vi "CRIO_TCPWriteState.vi"(6 "Curr State":T1, 8 "error in (no error)":errorcluster, 9 "Transition? in":bool, 10 "Connected?":bool, 11 "TCP Network Connection in":refnum<k5>) -> (0 "error out":errorcluster, 3 "TCP Network Connection out":refnum<k5>)   [LabVIEW 2017]
uses:
  CRIO_StateEnum.ctl
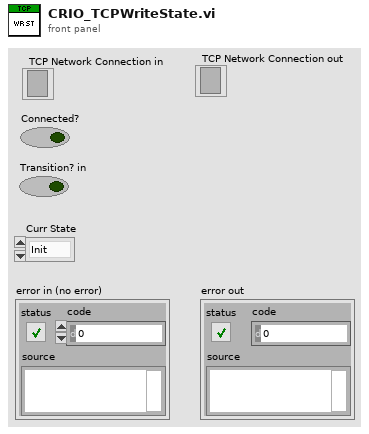
[diagram p1: front panel]
types:
  T1 = typedef "CRIO_StateEnum.ctl" = enum16{"Init", "Listen", "Wait", "Setup", "Ready to Launch", "Start Flight", "Accelerating", "Coasting", "Braking", "End Flight", "Loading", "Stop"}
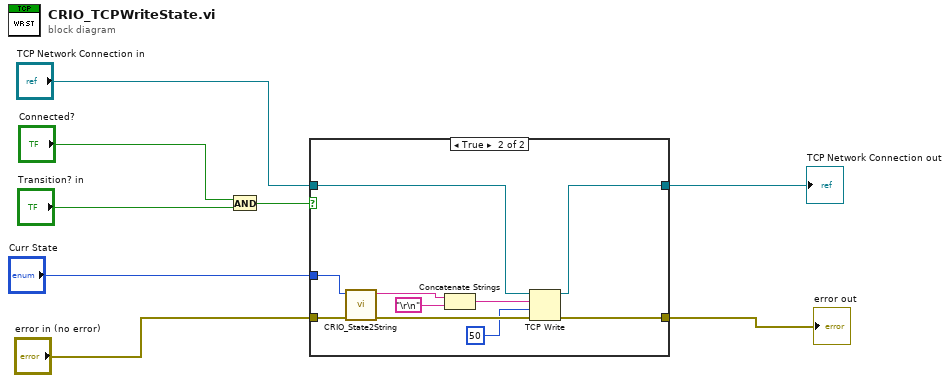
[diagram p0: block diagram]
diagram:
  n1 = And(x="Connected?", y="Transition? in") -> (x .and. y?=w2:bool)
  n2 = case shown="True" w2 {
    tunnel: [w9 w19] -> w3
    tunnel: "error in (no error)" -> [w9 w20]
    tunnel: "TCP Network Connection in" -> [w10 w16]
    tunnel: [w10 w17] -> w7
    tunnel: "Curr State" -> [_ w14]
    frame False {
    }
    frame True {
      n3 = call "CRIO_State2String.vi"("error in (no error)"=w20, "Curr State"=w14) -> ("error out"=w18:errorcluster, "State Str"=w13:string)  [unwired: 8 in]
      n4 = Concatenate Strings(w13, "\r\n") -> (w12:string)
      n5 = TCP Write(connection ID=w16, data in=w12, error in (no error)=w18, 9:50 ("timeout ms (25000)")) -> (connection ID out=w17:refnum<k5>, error out=w19:errorcluster)  [unwired: 1 out]
    }
  }
  "TCP Network Connection out" <- w7
  "error out" <- w3
